vi "THCD_401_Global.vi"() -> ()   [LabVIEW 2019]
panel:
  out "THCD401_FC2":dbl
  out "THCD401_FC1":dbl
  out "THCD401_ST":u32(colorbox)
  out "THCD401_FM1":dbl
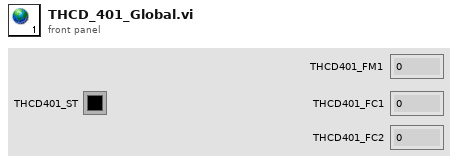
[diagram p1: front panel]
diagram:
